vi "串口选择.vi"() -> (3 "VISA resource name 2":refnum<visa-resource-name> caption="COM")   [LabVIEW 2018]
uses:
  <vilib>/Instr/_visa.llb/VISA Configure Serial Port (Instr).vi
panel:
  in  "VISA resource name":refnum<visa-resource-name>="COM11" caption="COM"
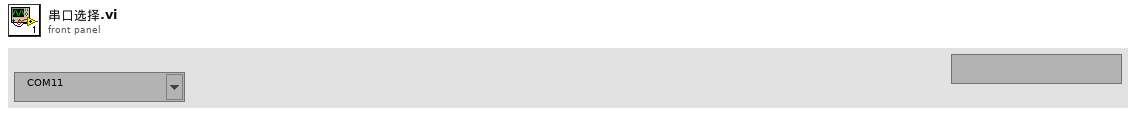
[diagram p1: front panel]
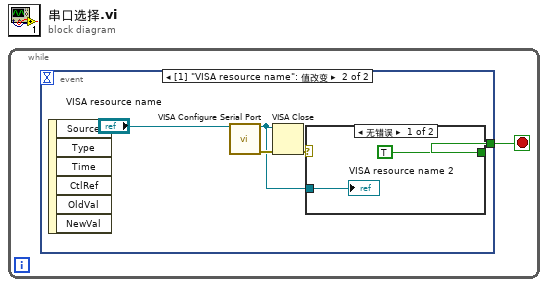
[diagram p0: block diagram]
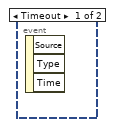
[diagram p2: hidden frame]
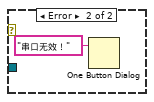
[diagram p3: hidden frame]
diagram:
  n1 = while {
    stop <- w1 stop-if-true
    n2 = event shown="[1] \"VISA resource name\": 值改变" {
      selector: _ -> [_ _]
      dyn-events: _ -> [_ _]
      timeout: _ -> [_ _]
      tunnel: [_ w3] -> w1
      event Timeout {
        n3 = event-data() -> ()  [unwired: 1 in, 3 out]
      }
      event "VISA resource name": Value Change {
        n4 = event-data() -> ()  [unwired: 1 in, 6 out]
        n5 = call-poly "VISA Configure Serial Port"("VISA resource name"="VISA resource name") -> ("VISA resource name out"=w2:refnum<visa-resource-name>, "error out"=w5:errorcluster)  [unwired: 13 in]
        n6 = VISA Close(VISA resource name=w2, error in (no error)=w5) -> (error out=w4:errorcluster)
        n7 = case shown="无错误" w4 {
          tunnel: [TRUE _] -> w3
          tunnel: w2 -> [w7 _]
          frame No Error {
            "VISA resource name 2" <- w7
          }
          frame Error {
            n8 = One Button Dialog(message="串口无效！" ("消息")) -> ()  [unwired: 1 in, 1 out]
          }
        }
      }
    }
  }
